vi "Sistem Kalkulasi Flowrate.vi"() -> ()   [LabVIEW 2014]
uses:
  <vilib>/Instr/_visa.llb/VISA Configure Serial Port (Instr).vi
panel:
  out "Flowrate Chart":dbl(graph)
  out "Flowrate":dbl
  in  "Table Control":string[][](table)
  out "Temperatur":dbl
  out "Differential Pressure":dbl
  out "Tekanan":dbl
  out "Tekanan":dbl
  out "read buffer":string
  in  "Port ARDUINO":refnum<visa-resource-name>
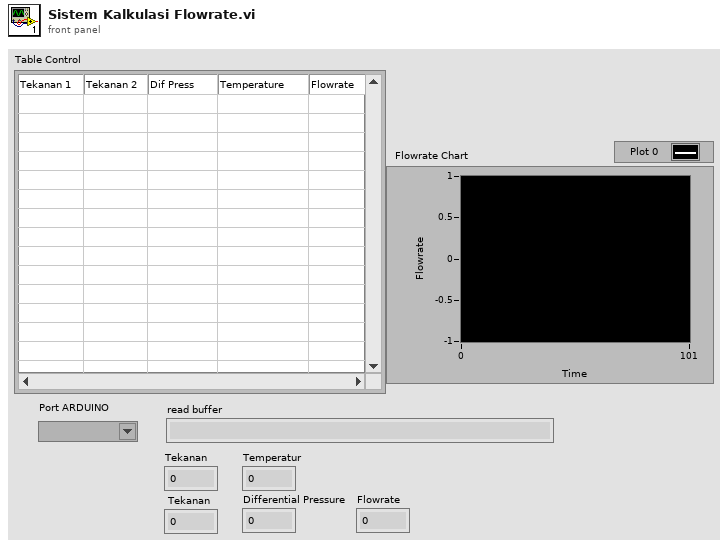
[diagram p1: front panel]
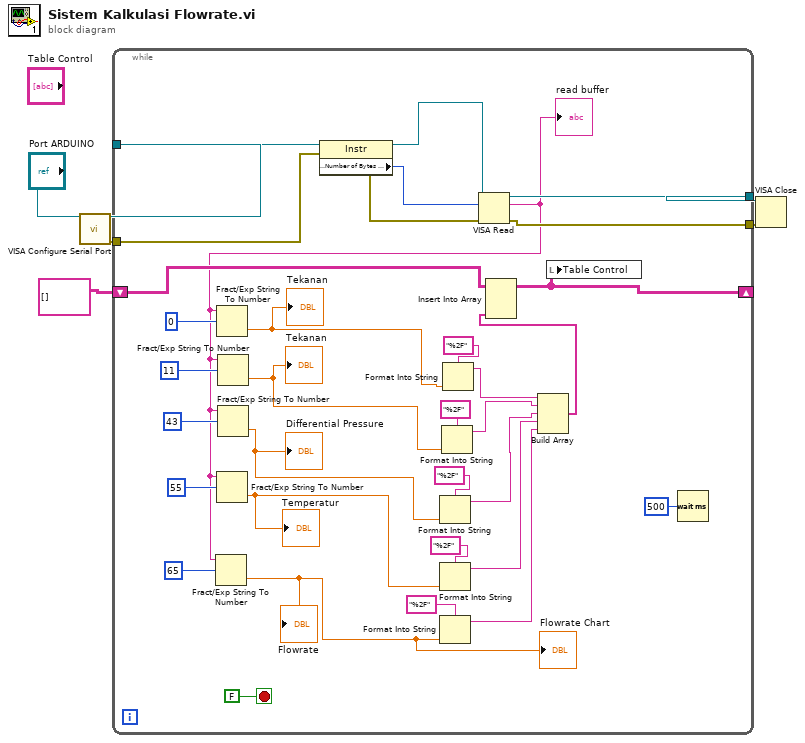
[diagram p0: block diagram]
diagram:
  n1 = call-poly "VISA Configure Serial Port"("VISA resource name"="Port ARDUINO") -> ("VISA resource name out"=w5:refnum<visa-resource-name>, "error out"=w4:errorcluster)  [unwired: 13 in]
  n2 = while {
    tunnel: w5 -> [w36]
    tunnel: w4 -> [w35]
    tunnel: [w34] -> w3
    tunnel: [w33] -> w2
    shift-right: [w14] -> _
    shift-left: string[][] [] -> [w15]
    stop <- FALSE stop-if-true
    n3 = property class="Instr"(reference=w36, error in=w35) -> (reference out=w38:refnum<visa-resource-name>, error out=w39:errorcluster, "Serial Settings:Number of Bytes at Serial Port"=w37:u32)
    n4 = VISA Read(VISA resource name=w38, byte count=w37, error in (no error)=w39) -> (VISA resource name out=w34:refnum<visa-resource-name>, read buffer=w13:string, error out=w33:errorcluster)  [unwired: 1 out]
    "read buffer" <- w13
    n5 = Fract/Exp String To Number(string=w13, offset=65) -> (number=w9:dbl)  [unwired: 2 in, 1 out]
    "Flowrate" <- w9
    "Flowrate Chart" <- w9
    n6 = Fract/Exp String To Number(string=w13, offset=0) -> (number=w19:dbl)  [unwired: 2 in, 1 out]
    "Tekanan" <- w19
    n7 = Fract/Exp String To Number(string=w13, offset=55) -> (number=w16:dbl)  [unwired: 2 in, 1 out]
    "Temperatur" <- w16
    n8 = Fract/Exp String To Number(string=w13, offset=11) -> (number=w18:dbl)  [unwired: 2 in, 1 out]
    "Tekanan" <- w18
    n9 = Fract/Exp String To Number(string=w13, offset=43) -> (number=w17:dbl)  [unwired: 2 in, 1 out]
    "Differential Pressure" <- w17
    n10 = Format Into String(format string="%2F", w17) -> (resulting string=w27:string)  [unwired: 2 in, 1 out]
    n11 = Format Into String(format string="%2F", w16) -> (resulting string=w28:string)  [unwired: 2 in, 1 out]
    n12 = Format Into String(format string="%2F", w9) -> (resulting string=w10:string)  [unwired: 2 in, 1 out]
    n13 = Format Into String(format string="%2F", w18) -> (resulting string=w26:string)  [unwired: 2 in, 1 out]
    n14 = Format Into String(format string="%2F", w19) -> (resulting string=w25:string)  [unwired: 2 in, 1 out]
    n15 = Build Array(w25, w26, w27, w28, w10) -> (w23:string[])
    n16 = Insert Into Array(array=w15, new element=w23) -> (w14:string[][])  [unwired: 2 in]
    n17 = local write "Table Control"(w14) -> ()
    n18 = Wait (ms)(milliseconds to wait=u32 500) -> ()  [unwired: 1 out]
  }
  n19 = VISA Close(VISA resource name=w3, error in (no error)=w2) -> ()  [unwired: 1 out]
